vi "2D String to 1D DBL.vi"(10 "Column":i32=1, 11 "Data Table":string[][](array[string])) -> (3 "DBL Column":dbl[](array[numeric]))   [LabVIEW 2013]
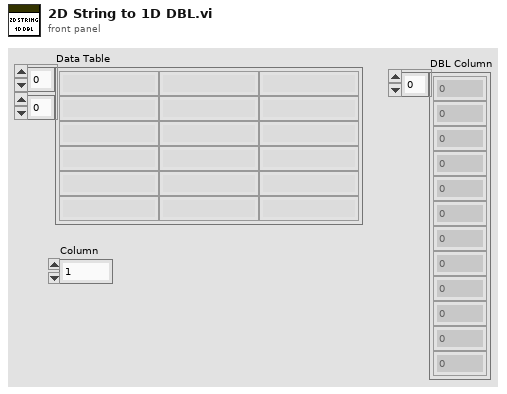
[diagram p1: front panel]
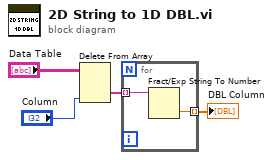
[diagram p0: block diagram]
diagram:
  n1 = Delete From Array(array="Data Table", index (col)="Column") -> (deleted portion=w2:string[])  [unwired: 2 in, 1 out]
  n2 = for {
    tunnel: w2 -> [w6] mode=indexing
    tunnel: [w5] -> w1 mode=indexing
    n3 = Fract/Exp String To Number(string=w6) -> (number=w5:dbl)  [unwired: 3 in, 1 out]
  }
  "DBL Column" <- w1
